vi "Serialize LabVIEW Object to JSON.vi"() -> ()   [LabVIEW 2020]
doc: "This VI demonstrates a function of the GCraftsman JSON Serialization Toolkit.\n\nIt uses the 'Flatten to JSON String' function to serialize LabVIEW objects to JSON format, including hierarchical and composite relationships.\n\nThis does not require the classes to have accessor methods.\n\nGCraftsman JSON Object Serialization Toolkit\nwww.GCraftsman.com\nCopyright (c) 2017, GCraftsman"
uses:
  Class2/Class2.lvclass
  Class3/Class3.lvclass
  library/JKI JSON Object Serialization.lvlib
panel:
  out "JSON String":string
  in  "myBool":bool=TRUE
  in  "anotherNumber":dbl=123.0 format="%#_13g"
  in  "someNumber":dbl=456.0 format="%#_13g"
  in  "myNum 2":dbl=555.0 format="%#_13g"
  in  "myNum":dbl=444.0 format="%#_13g"
  # "This VI demonstrates a function of the GCraftsman JSON Serialization Toolkit.\n\nLook at the block diagram to see that the 'Flatten to JSON String' function can serialize LabVIEW objects, including hierarchical and composite relationships.\n\nRun this VI to see the output JSON string."
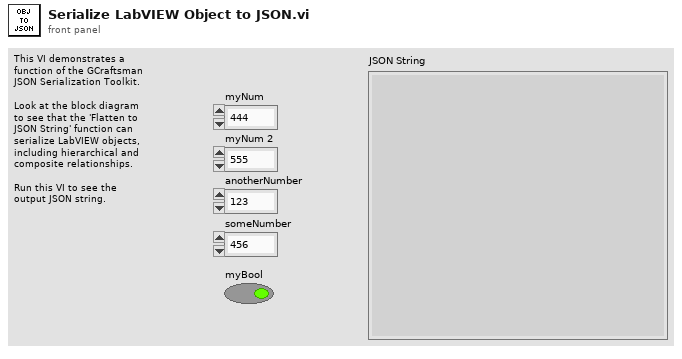
[diagram p1: front panel]
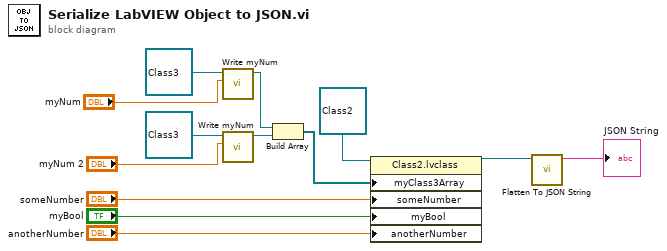
[diagram p0: block diagram]
diagram:
  n1 = call-dynamic "Write myNum.vi"("myNum"="myNum", "Test3 in"=refnum<class "Class3.lvclass"> refnum ("Test3.lvclass")) -> ("Test3 out"=w8:refnum<class "Class3.lvclass">)  [unwired: 8 in, 1 out]
  n2 = call-dynamic "Write myNum.vi"("myNum"="myNum 2", "Test3 in"=refnum<class "Class3.lvclass"> refnum ("Test3.lvclass")) -> ("Test3 out"=w11:refnum<class "Class3.lvclass">)  [unwired: 8 in, 1 out]
  n3 = Build Array(w8, w11) -> (w6:refnum<class "Class3.lvclass">[])
  n4 = property class="Class2.lvclass"(reference=refnum<class "Class2.lvclass"> refnum ("Test2.lvclass"), "myClass3Array"=w6, "someNumber"="someNumber", "myBool"="myBool", "anotherNumber"="anotherNumber") -> (reference out=w2:refnum<class "Class2.lvclass">)  [unwired: 1 in, 1 out]
  n5 = call "Flatten To JSON String.vi"("Variant"=w2) -> ("JSON String"=→"JSON String":string)  [unwired: 9 in, 1 out]
